vi "User Interface.vi"(10 "Test File Path":path=path "") -> ()   [LabVIEW 2020, in "Execution UI.lvclass"]
uses:
  Execution UI.lvclass
  Execution UI.lvclass/Execution UI.ctl
  Helper Classes/Test Tree/Test Tree.lvclass
  Helper Classes/Test Result Tree/Test Result Tree.lvclass
  Result Classes/Test Case Result/Test Case Result.lvclass
  Result Classes/Method Result/Method Result.lvclass
  Result Classes/Test Suite Result/Test Suite Result.lvclass
  Application Framework/Process Classes/Process/Process.lvclass
  Application Framework/Process Classes/Error Handler/Error Handler.lvclass
  <vilib>/Utility/miscctls.llb/LVNodeAndColumnTypeDef.ctl
  Test Runner/Test Runner.lvclass
  Private/TypeDefs/Execution State.ctl
  Helper Classes/Buffered Test Finder/Indexing Test Finder.lvclass
  Helper Classes/Result Table/Result Table/Result Table.lvclass
  Report Generator/Report Generator.lvclass
  Result Classes/Result View/Result View.vi
  Test Result View/Test Result View.lvclass
  Helper Classes/Test Finder/Test Finder.lvclass
  Execution Profiler/Execution Profiler.lvclass
  <vilib>/Platform/browser.llb/Open URL in Default Browser (string).vi
  Coverage Analyzer Process/Coverage Analyzer Process.lvclass
  C:/Git/astemes-lunit/source/Framework/Helper Classes/Test Tree/Test Tree.lvclass
  C:/Git/astemes-lunit/source/Framework/Helper Classes/Test Result Tree/Test Result Tree.lvclass
  C:/Git/astemes-lunit/source/Application Framework/Process Classes/Process/Process.lvclass
  C:/Git/astemes-lunit/source/Framework/Execution UI/Execution UI.lvclass
  C:/Git/astemes-lunit/source/Framework/Helper Classes/Test Finder/Test Finder.lvclass
  C:/Git/astemes-lunit/source/Framework/Helper Classes/Buffered Test Finder/Indexing Test Finder.lvclass
  C:/Git/astemes-lunit/source/Framework/Execution Profiler/Execution Profiler.lvclass
  C:/Git/astemes-lunit/source/Framework/Coverage Analyzer Process/Coverage Analyzer Process.lvclass
panel:
  in  "Refresh":bool
  in  "Run Single Test":bool
  in  "Stop":bool
  in  "Run All Tests":bool
  in  "Eject":bool
  in  "Save":bool
  in  "Collapse":bool
  in  "Expand":bool
  out "Progress bar":dbl(slide) scale=0.0..100.0
  out "Results":i32(listbox)=-1
  in  "Test Results":string[](tree)
  in  "Filter fails":bool
  out "Description":string
  out "Status":string
  out "error out":errorcluster
  in  "error in (no error)":errorcluster
  # "1"
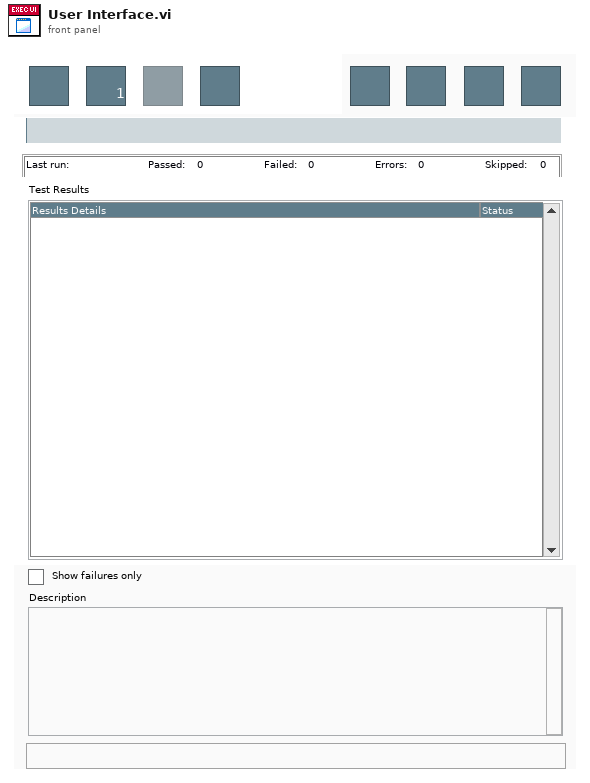
[diagram p1: front panel]
types:
  T1 = cluster{"Event Registration Refnum":refnum<event-registration>, "Event Registration Refnum":refnum<event-registration>, "Event Registration Refnum":refnum<event-registration>}
  T2 = typedef "LVNodeAndColumnTypeDef.ctl" = cluster{"Node":string, "Column":i32}
  T3 = enum32{"Invalid", "Standard", "Closed", "Hidden", "Minimized", "Maximized"}
  T4 = typedef "Execution UI.lvclass/Execution State.ctl" = enum16{"Idle", "Running"}
  T5 = enum8{"Enabled", "Disabled", "Disabled and Grayed Out"}
  T6 = typedef "Assertion Result.lvclass/Status.ctl" = enum16{"Pass", "Fail", "Error", "Skipped", "Setup Error", "Broken", "Teardown Error"}
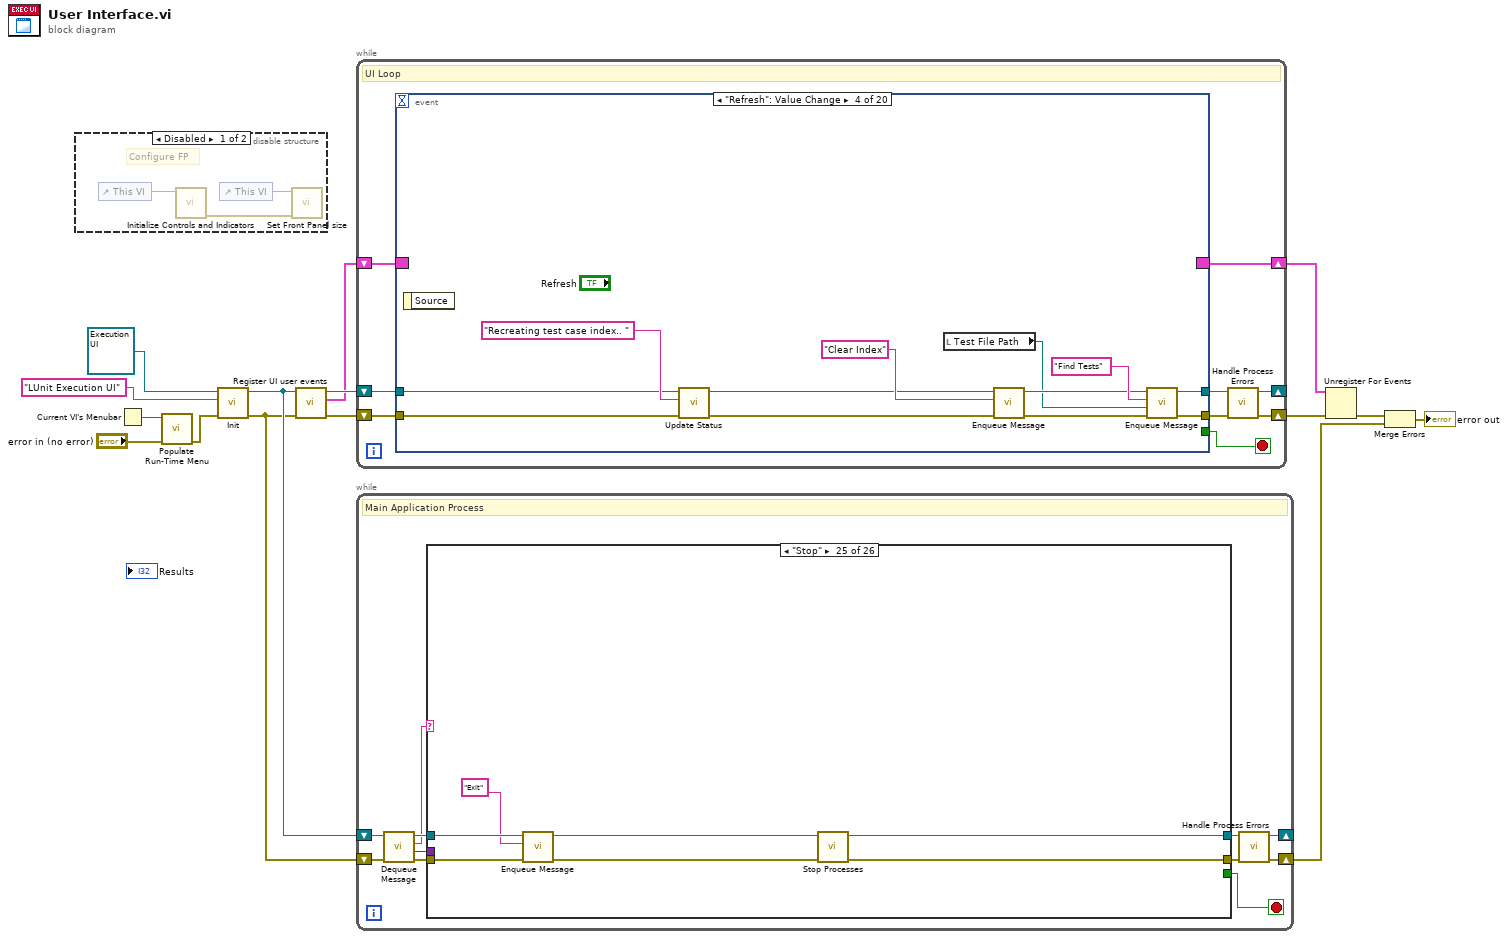
[diagram p0: block diagram]
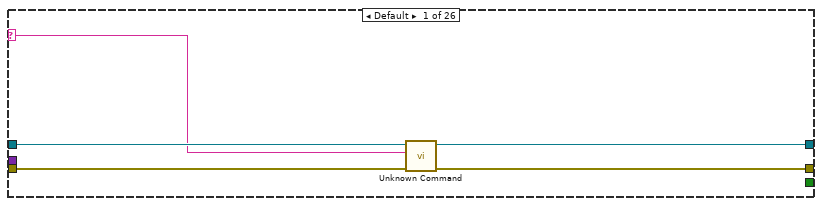
[diagram p2: hidden frame]
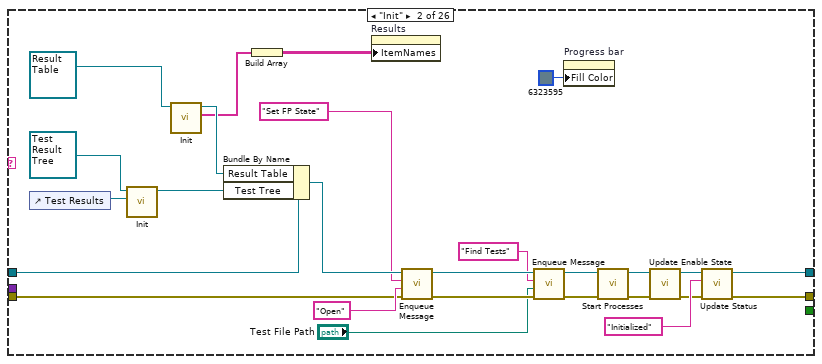
[diagram p3: hidden frame]
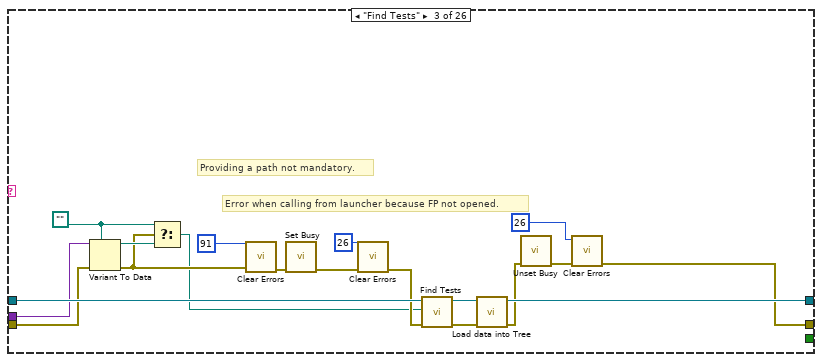
[diagram p4: hidden frame]
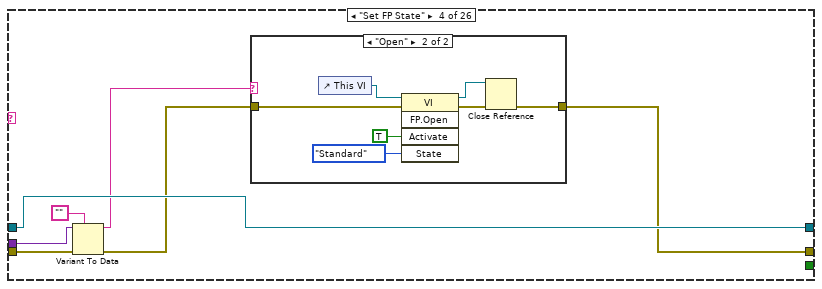
[diagram p5: hidden frame]
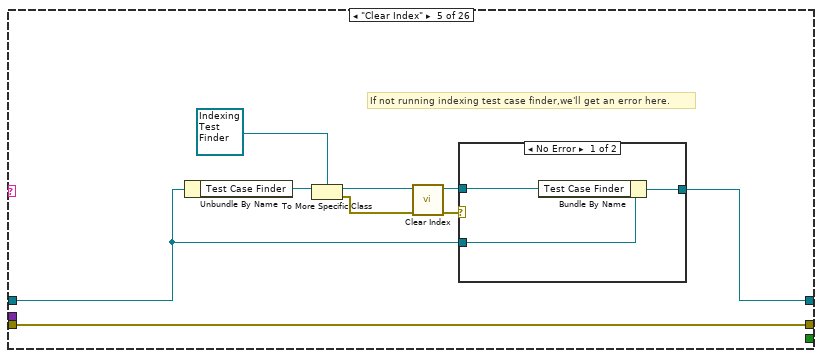
[diagram p7: hidden frame]
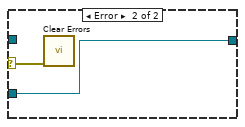
[diagram p8: hidden frame]
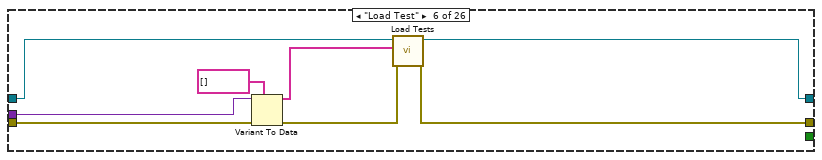
[diagram p9: hidden frame]
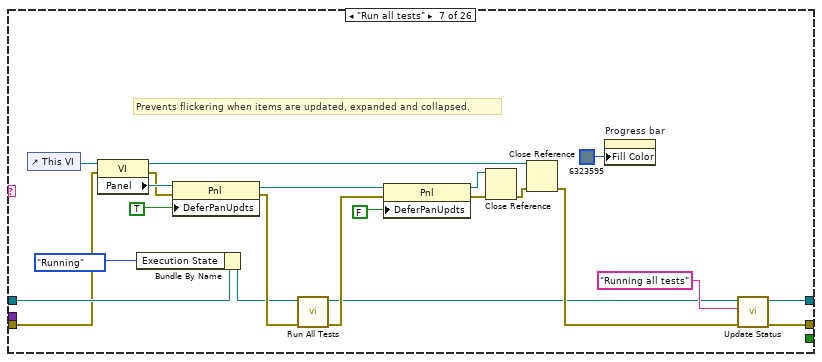
[diagram p10: hidden frame]
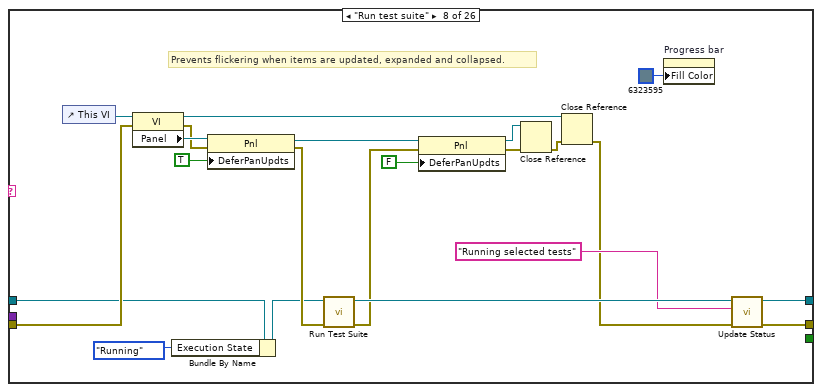
[diagram p11: hidden frame]
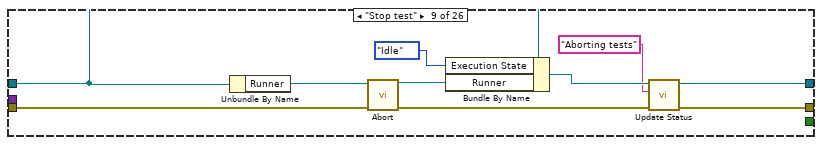
[diagram p12: hidden frame]
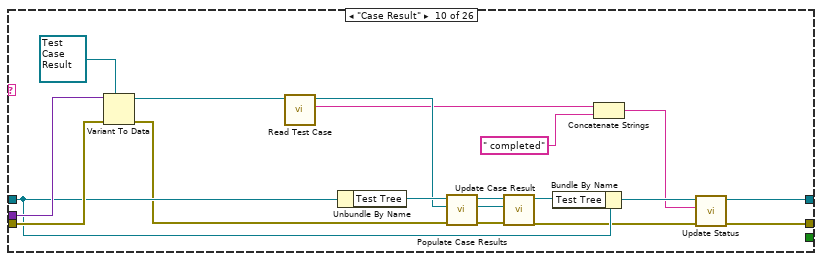
[diagram p13: hidden frame]
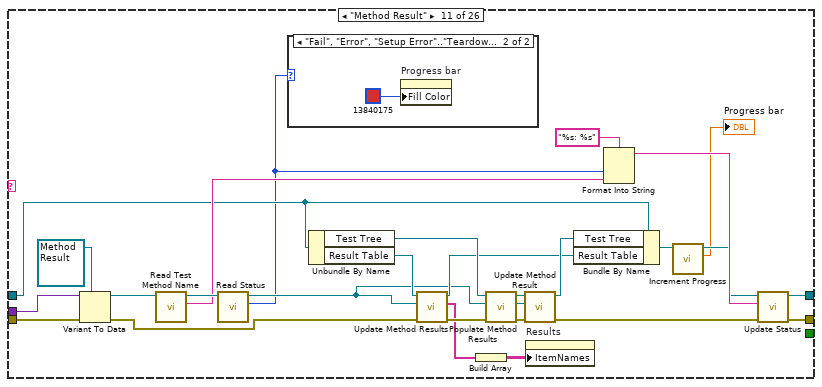
[diagram p14: hidden frame]
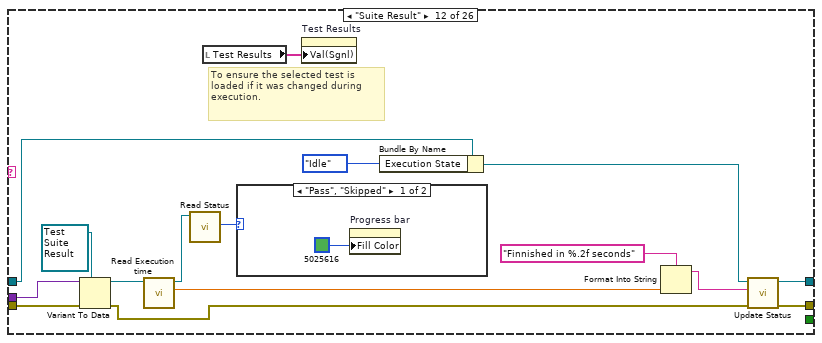
[diagram p16: hidden frame]
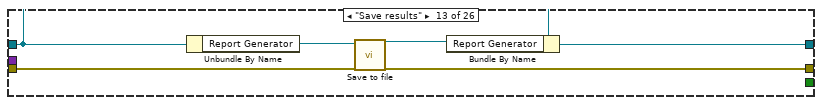
[diagram p18: hidden frame]
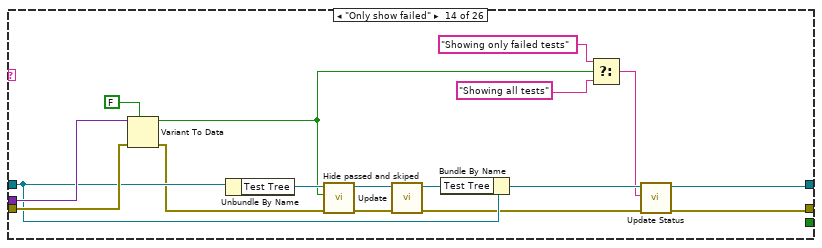
[diagram p19: hidden frame]
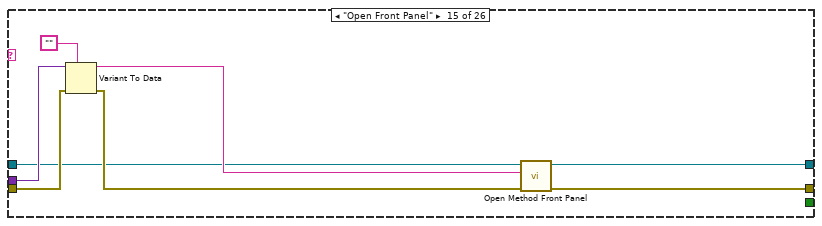
[diagram p20: hidden frame]
diagram:
  n1 = disable-structure shown="Disabled" {
    frame Disabled {
      # "Configure FP"
      n2 = control-ref of="This VI"() -> (w17:refnum<vi>)
      n3 = call "Initialize Controls and Indicators.vi"("VI in"=w17) -> ("error out"=w16:errorcluster)  [unwired: 10 in]
      n4 = control-ref of="This VI"() -> (w18:refnum<vi>)
      n5 = call "Set Front Panel size.vi"("error in (no error)"=w16, "VI in"=w18) -> ()  [unwired: 9 in, 1 out]
    }
    frame Enabled {
    }
  }
  n6 = Current VI's Menubar() -> (w1:refnum<k9>)
  n7 = call "Populate Run-Time Menu.vi"("error in (no error)"="error in (no error)", "Menu in"=w1) -> ("error out"=w2:errorcluster)  [unwired: 9 in]
  n8 = call-dynamic "Init.vi"("error in (no error)"=w2, "Name"="LUnit Execution UI", "Execution UI In"=refnum<class "Execution UI.lvclass"> refnum ("Test Execution UI.lvclass")) -> ("error out"=w7:errorcluster, "Execution UI Out"=w8:refnum<class "Execution UI.lvclass">)  [unwired: 7 in]
  n9 = call "Register UI user events.vi"("error in (no error)"=w7, "Execution UI In"=w8) -> ("error out"=w14:errorcluster, "output cluster"=w12:T1, "Execution UI Out"=w15:refnum<class "Execution UI.lvclass">)  [unwired: 7 in]
  n10 = while {
    shift-right: [w19] -> w6
    shift-left: w14 -> [w26]
    shift-right: [w21] -> _
    shift-left: w15 -> [w27]
    shift-right: [w23] -> w13
    shift-left: w12 -> [w22]
    stop <- w24 stop-if-true
    # "UI Loop"
    n11 = event shown="[3] \"Refresh\": Value Change" {
      selector: w22 -> [_ _ _ _ _ _ _ _ _ _ _ _ _ _ _ _ _ _ _ _]
      dyn-events: [_ _ _ _ _ _ _ _ _ _ _ _ _ _ _ _ _ _ _ _] -> w23
      timeout: _ -> [_ _ _ _ _ _ _ _ _ _ _ _ _ _ _ _ _ _ _ _]
      tunnel: w27 -> [w33 w36 w43 w47 w59 w69 w94 w101 w111 w116 w120 w130 w141 w149 w184 w305 w311 w312 w318 w326]
      tunnel: w26 -> [w34 w37 w41 w45 w61 w70 w96 w104 w110 w114 w118 w129 w131 w142 w183 w303 w309 w313 w320 w323]
      tunnel: [w34 w37 w40 w54 w58 w68 w93 w100 w108 w113 w119 w128 w132 w147 w182 w302 w308 w313 w317 w324] -> w20
      tunnel: [w33 w36 w42 w55 w56 w67 w91 w98 w109 w115 w121 w127 w141 w146 w181 w304 w310 w312 w315 w325] -> w25
      tunnel: [_ _ _ _ _ _ _ _ _ _ _ _ _ _ _ _ _ TRUE _ _] -> w24
      event "Collapse": Value Change {
        n12 = event-data() -> ()  [unwired: 1 in, 6 out]
        n13 = property on="Test Results" class="Tree (strict)"() -> ("All Tags"=w31:string[])  [unwired: 2 in, 2 out]
        n14 = invoke on="Test Results" class="Tree (strict)" method="Open/Close.Open/Close All"("Open"=FALSE ("Open?")) -> ()  [unwired: 3 in, 4 out]
        n15 = Index Array(array=w31) -> (element=w28:string)  [unwired: 1 in]
        n16 = Bundle By Name(cluster=T2 {"Node"="", "Column"=0} ("Top Left Visible Cell"), "Node"=w28) -> (w29:T2)
        n17 = property on="Test Results" class="Tree (strict)"("TopLeft"=w29) -> ()  [unwired: 2 in, 2 out]
      }
      event "Expand": Value Change {
        n18 = event-data() -> ()  [unwired: 1 in, 6 out]
        n19 = invoke on="Test Results" class="Tree (strict)" method="Open/Close.Open/Close All"("Open"=TRUE ("Open?")) -> ()  [unwired: 3 in, 4 out]
      }
      event "Filter fails": Value Change {
        n20 = event-data() -> ()  [unwired: 1 in, 1 out]
        n21 = call "Enqueue Message.vi"("error in (no error)"=w41, "Message Data"="Filter fails", "Message"="Only show failed", "Process In"=w43) -> ("error out"=w40:errorcluster, "Process Out"=w42:refnum<class "Execution UI.lvclass">)  [unwired: 6 in]
      }
      event "Refresh": Value Change {
        n22 = event-data() -> ()  [unwired: 1 in, 1 out]
        n23 = call "Update Status.vi"("error in (no error)"=w45, "Status"="Recreating test case index.. ", "Execution UI In"=w47) -> ("error out"=w46:errorcluster, "Execution UI Out"=w48:refnum<class "Execution UI.lvclass">)  [unwired: 7 in]
        n24 = local read "Test File Path"() -> (w44:path)
        n25 = call "Enqueue Message.vi"("error in (no error)"=w46, "Message"="Clear Index", "Process In"=w48) -> ("error out"=w51:errorcluster, "Process Out"=w52:refnum<class "Execution UI.lvclass">)  [unwired: 7 in]
        n26 = call "Enqueue Message.vi"("error in (no error)"=w51, "Message Data"=w44, "Message"="Find Tests", "Process In"=w52) -> ("error out"=w54:errorcluster, "Process Out"=w55:refnum<class "Execution UI.lvclass">)  [unwired: 6 in]
      }
      event "Run All Tests": Value Change {
        w60 = "Run all tests"  # Message
        n27 = event-data() -> ()  [unwired: 1 in, 1 out]
        n28 = call "Enqueue Message.vi"("error in (no error)"=w61, "Message"=w60, "Process In"=w59) -> ("error out"=w62:errorcluster, "Process Out"=w57:refnum<class "Execution UI.lvclass">)  [unwired: 7 in]
        n29 = call "Update Enable State.vi"("error in (no error)"=w62, "Execution UI In"=w57) -> ("error out"=w58:errorcluster, "Execution UI Out"=w56:refnum<class "Execution UI.lvclass">)  [unwired: 8 in]
      }
      event Key Down {
        # "Run all tests on ctrl+r"
        n30 = event-data() -> ("Char"=w63:i16, "PlatMods.Ctrl"=w66:bool, "PlatMods.Opt"=w65:bool)  [unwired: 1 in]
        n31 = Or(x=w66, y=w65) -> (x .or. y?=w64:bool)
        n32 = case "CTRL" shown="True" w64 {
          tunnel: w70 -> [w71 w77]
          tunnel: w69 -> [w72 w76]
          tunnel: [w71 w75] -> w68
          tunnel: [w72 w74] -> w67
          tunnel: w63 -> [_ w73]
          frame False {
          }
          frame True {
            n33 = case "Key" shown="119" w73 {
              tunnel: w77 -> [w78 w85 w89]
              tunnel: w76 -> [w79 w83 w90]
              tunnel: [w78 w82 w87] -> w75
              tunnel: [w79 w80 w88] -> w74
              frame Default {
              }
              frame 114 {
                w84 = "Run all tests"  # Message
                # "R"
                n34 = call "Enqueue Message.vi"("error in (no error)"=w85, "Message"=w84, "Process In"=w83) -> ("error out"=w86:errorcluster, "Process Out"=w81:refnum<class "Execution UI.lvclass">)  [unwired: 7 in]
                n35 = call "Update Enable State.vi"("error in (no error)"=w86, "Execution UI In"=w81) -> ("error out"=w82:errorcluster, "Execution UI Out"=w80:refnum<class "Execution UI.lvclass">)  [unwired: 8 in]
              }
              frame 119 {
                # "W"
                n36 = call-dynamic "Stop.vi"("error in (no error)"=w89, "Execution UI In"=w90) -> ("error out"=w87:errorcluster, "Execution UI Out"=w88:refnum<class "Execution UI.lvclass">)  [unwired: 7 in, 1 out]
              }
            }
          }
        }
      }
      event "Run Single Test": Value Change {
        w95 = "Run test suite"  # Message
        n37 = event-data() -> ()  [unwired: 1 in, 1 out]
        n38 = call "Enqueue Message.vi"("error in (no error)"=w96, "Message"=w95, "Process In"=w94) -> ("error out"=w97:errorcluster, "Process Out"=w92:refnum<class "Execution UI.lvclass">)  [unwired: 7 in]
        n39 = call "Update Enable State.vi"("error in (no error)"=w97, "Execution UI In"=w92) -> ("error out"=w93:errorcluster, "Execution UI Out"=w91:refnum<class "Execution UI.lvclass">)  [unwired: 8 in]
      }
      event "Stop": Value Change {
        n40 = event-data() -> ()  [unwired: 1 in, 2 out]
        n41 = call "Enqueue Message.vi"("error in (no error)"=w104, "Message"="Stop test", "Process In"=w101) -> ("error out"=w103:errorcluster, "Process Out"=w99:refnum<class "Execution UI.lvclass">)  [unwired: 7 in]
        n42 = call "Update Enable State.vi"("error in (no error)"=w103, "Execution UI In"=w99) -> ("error out"=w100:errorcluster, "Execution UI Out"=w98:refnum<class "Execution UI.lvclass">)  [unwired: 8 in]
      }
      event "Test Results": Double Click {
        n43 = event-data() -> ("Tag"=w106:string)  [unwired: 1 in]
        n44 = To Variant(anything=w106) -> (Variant=w105:variant)
        n45 = call "Enqueue Message.vi"("error in (no error)"=w110, "Message Data"=w105, "Message"="Open Front Panel", "Process In"=w111) -> ("error out"=w108:errorcluster, "Process Out"=w109:refnum<class "Execution UI.lvclass">)  [unwired: 6 in]
      }
      event "Save": Value Change {
        n46 = event-data() -> ()  [unwired: 1 in, 4 out]
        n47 = call "Enqueue Message.vi"("error in (no error)"=w114, "Message"="Save results", "Process In"=w116) -> ("error out"=w113:errorcluster, "Process Out"=w115:refnum<class "Execution UI.lvclass">)  [unwired: 7 in]
      }
      event "Eject": Value Change {
        n48 = event-data() -> ()  [unwired: 1 in, 4 out]
        n49 = call "Enqueue Message.vi"("error in (no error)"=w118, "Message"="Launch Results View", "Process In"=w120) -> ("error out"=w119:errorcluster, "Process Out"=w121:refnum<class "Execution UI.lvclass">)  [unwired: 7 in]
      }
      event "Test Results": Value Change {
        n50 = event-data() -> ("NewVal"=w122:string[])  [unwired: 1 in]
        n51 = call "Enqueue Message.vi"("error in (no error)"=w129, "Message Data"=w122, "Message"="Update Description", "Process In"=w130) -> ("error out"=w126:errorcluster, "Process Out"=w125:refnum<class "Execution UI.lvclass">)  [unwired: 6 in]
        n52 = call "Enqueue Message.vi"("error in (no error)"=w126, "Message Data"=w122, "Message"="Load Test", "Process In"=w125) -> ("error out"=w128:errorcluster, "Process Out"=w127:refnum<class "Execution UI.lvclass">)  [unwired: 6 in]
      }
      event Pane Size {
        # "Set column sizes on pane resize."
        n53 = event-data() -> ()  [unwired: 1 in, 1 out]
        n54 = property on="Test Results" class="Tree (strict)"(error in=w131) -> (error out=w133:errorcluster, "Width"=w134:u32)  [unwired: 1 in, 1 out]
        n55 = Quotient & Remainder(x=w134, y=u32 10) -> (floor(x/y)=w138:u32)  [unwired: 1 out]
        n56 = Multiply(x=w138, y=u32 8) -> (x*y=w135:u32)
        n57 = property on="Test Results" class="Tree (strict)"(error in=w133, "ActiveColNum"=0 ("Active Cell:Active Column Number"), "Width"=w135, "ActiveColNum"=1 ("Active Cell:Active Column Number"), "Width"=w135) -> (error out=w132:errorcluster)  [unwired: 1 in, 1 out]
      }
      event "Test File Path": Value Change {
        # "This case is triggered when running test cases through VI Server.\nTo control test execution from an external VI - get a reference to the \"Test File Path\" control on the User Interface.vi and update the value with the path to test case using a property node."
        n58 = event-data() -> ("NewVal"=w148:path)  [unwired: 1 in]
        n59 = call <vilib>:"Get File Extension.vi"("error in (no error)"=w142, "file"=w148) -> ("error out"=w143:errorcluster, "lowercase file extension"=w144:string, "dup file"=w145:path)  [unwired: 5 in, 2 out]
        n60 = case shown="Default" w144 {
          tunnel: w149 -> [w151 w170 w179]
          tunnel: w143 -> [w150 w169 w178]
          tunnel: w145 -> [_ w164 w176]
          tunnel: [w150 w156 w173] -> w147
          tunnel: [w151 w154 w172] -> w146
          frame Default {
          }
          frame "lvclass" {
            n61 = call "Enqueue Message.vi"("error in (no error)"=w169, "Message Data"=w164, "Message"="Find Tests", "Process In"=w170) -> ("error out"=w160:errorcluster, "Process Out"=w162:refnum<class "Execution UI.lvclass">)  [unwired: 6 in]
            n62 = call <vilib>:"Get LV Class Default Value.vi"("error in (no error)"=w160, "class path"=w164) -> ("error out"=w166:errorcluster, "object"=w165:refnum<class>)  [unwired: 8 in]
            n63 = call <vilib>:"Get LV Class Name.vi"("error in (no error)"=w166, "object"=w165) -> ("error out"=w159:errorcluster, "class name"=w153:string)  [unwired: 8 in]
            n64 = Build Array(w153) -> (w158:string[])
            n65 = call "Enqueue Message.vi"("error in (no error)"=w159, "Message Data"=w158, "Message"="Load Test", "Process In"=w162) -> ("error out"=w163:errorcluster, "Process Out"=w161:refnum<class "Execution UI.lvclass">)  [unwired: 6 in]
            n66 = call "Enqueue Message.vi"("error in (no error)"=w163, "Message"="Run test suite", "Process In"=w161) -> ("error out"=w157:errorcluster, "Process Out"=w155:refnum<class "Execution UI.lvclass">)  [unwired: 7 in]
            n67 = call "Enqueue Message.vi"("error in (no error)"=w157, "Message Data"=w153, "Message"="Set Top Left Tree Node", "Process In"=w155) -> ("error out"=w156:errorcluster, "Process Out"=w154:refnum<class "Execution UI.lvclass">)  [unwired: 6 in]
          }
          frame "lvproj" {
            n68 = call "Enqueue Message.vi"("error in (no error)"=w178, "Message Data"=w176, "Message"="Find Tests", "Process In"=w179) -> ("error out"=w174:errorcluster, "Process Out"=w175:refnum<class "Execution UI.lvclass">)  [unwired: 6 in]
            n69 = call "Enqueue Message.vi"("error in (no error)"=w174, "Message"="Run all tests", "Process In"=w175) -> ("error out"=w173:errorcluster, "Process Out"=w172:refnum<class "Execution UI.lvclass">)  [unwired: 7 in]
          }
        }
      }
      event Menu Selection (User) {
        n70 = event-data() -> ("ItemTag"=w185:string)  [unwired: 1 in]
        n71 = case shown="\"Coverage Analyzer...\"" w185 {
          tunnel: w184 -> [w199 w201 w208 w223 w226 w238 w255 w268 w272 w277 w285 w289 w293 w294 w299]
          tunnel: w183 -> [w186 w200 w209 w224 w227 w235 w252 w270 w276 w281 w282 w286 w290 w295 w298]
          tunnel: [w187 w200 w210 w221 w228 w236 w253 w269 w274 w279 w283 w287 w291 w295 w297] -> w182
          tunnel: [w199 w201 w211 w220 w229 w237 w254 w268 w273 w278 w285 w289 w293 w294 w296] -> w181
          frame "Full size" {
            # "This is the same as done in event case for Result Pane: Pane Size, but that case is not trigerd on maximizing window."
            n72 = control-ref of="This VI"() -> (w198:refnum<vi>)
            n73 = property on="Property Node" class="VI"(reference=w198, error in=w186, "FP.State"=T3."Maximized" ("Front Panel Window:State")) -> (error out=w189:errorcluster)  [unwired: 1 out]
            n74 = property on="Test Results" class="Tree (strict)"(error in=w189) -> (error out=w188:errorcluster, "Width"=w196:u32)  [unwired: 1 in, 1 out]
            n75 = Quotient & Remainder(x=w196, y=u32 10) -> (floor(x/y)=w195:u32)  [unwired: 1 out]
            n76 = Multiply(x=w195, y=u32 7) -> (x*y=w194:u32)
            n77 = property on="Test Results" class="Tree (strict)"(error in=w188, "ActiveColNum"=0 ("Active Cell:Active Column Number"), "Width"=w194, "ActiveColNum"=1 ("Active Cell:Active Column Number"), "Width"=w194) -> (error out=w187:errorcluster)  [unwired: 1 in, 1 out]
          }
          frame Default {
          }
          frame "Open Project or Test class" {
            n78 = call "File Dialog"("prompt"="Please select a test class or project file to load.", "pattern (all files)"="*.lvclass;*.lvproj;*.lvlib", "pattern label"="Project or class") -> ("selected path"=w207:path, "cancelled"=w203:bool, "error out"=w202:errorcluster)  [unwired: 9 in, 1 out]
            n79 = call <vilib>:"Clear Errors.vi"("error in (no error)"=w202) -> ()  [unwired: 5 in, 2 out]
            n80 = case shown="False" w203 {
              tunnel: [w213 w219] -> w211
              tunnel: [w212 w218] -> w210
              tunnel: w209 -> [w212 w217]
              tunnel: w208 -> [w213 w216]
              tunnel: w207 -> [_ w215]
              frame True {
              }
              frame False {
                n81 = call "Enqueue Message.vi"("error in (no error)"=w217, "Message Data"=w215, "Message"="Find Tests", "Process In"=w216) -> ("error out"=w218:errorcluster, "Process Out"=w219:refnum<class "Execution UI.lvclass">)  [unwired: 6 in]
              }
            }
          }
          frame "Configure Test Runner" {
            n82 = Unbundle By Name(w223) -> ("Runner"=w225:refnum<class "Test Runner.lvclass">)
            n83 = call "Configure Test Runner.vi"("error in (no error)"=w224, "Report Generator In"=w225) -> ("error out"=w221:errorcluster, "Report Generator Out"=w222:refnum<class "Test Runner.lvclass">)  [unwired: 8 in]
            n84 = Bundle By Name(cluster=w223, "Runner"=w222) -> (w220:refnum<class "Execution UI.lvclass">)
          }
          frame "Configure Reporting" {
            n85 = Unbundle By Name(w226) -> ("Report Generator"=w231:refnum<class "Report Generator.lvclass">)
            n86 = call "Configure Report Generator.vi"("error in (no error)"=w227, "Report Generator In"=w231) -> ("error out"=w228:errorcluster, "Report Generator Out"=w230:refnum<class "Report Generator.lvclass">)  [unwired: 8 in]
            n87 = Bundle By Name(cluster=w226, "Report Generator"=w230) -> (w229:refnum<class "Execution UI.lvclass">)
          }
          frame "Execution Profiler..." {
            n88 = Current VI's Menubar() -> (w233:refnum<k9>)
            n89 = Get Menu Item Info(7:"Execution Profiler...", 11:w233) -> (4:w234:bool)  [unwired: 1 in, 6 out]
            n90 = case shown="False" w234 {
              tunnel: w238 -> [w243 w248]
              tunnel: [w242 w247] -> w237
              tunnel: [w241 w246] -> w236
              tunnel: w235 -> [w240 w245]
              frame False {
                n91 = call "Enqueue Message.vi"("error in (no error)"=w240, "Message"="Enable Execution Profiler", "Process In"=w243) -> ("error out"=w241:errorcluster, "Process Out"=w242:refnum<class "Execution UI.lvclass">)  [unwired: 7 in]
              }
              frame True {
                n92 = call "Enqueue Message.vi"("error in (no error)"=w245, "Message"="Disable Execution Profiler", "Process In"=w248) -> ("error out"=w246:errorcluster, "Process Out"=w247:refnum<class "Execution UI.lvclass">)  [unwired: 7 in]
              }
            }
          }
          frame "Coverage Analyzer..." {
            n93 = Current VI's Menubar() -> (w250:refnum<k9>)
            n94 = Get Menu Item Info(7:"Coverage Analyzer...", 11:w250) -> (4:w251:bool)  [unwired: 1 in, 6 out]
            n95 = case shown="True" w251 {
              tunnel: w255 -> [w260 w265]
              tunnel: [w259 w264] -> w254
              tunnel: [w258 w263] -> w253
              tunnel: w252 -> [w257 w262]
              frame False {
                n96 = call "Enqueue Message.vi"("error in (no error)"=w257, "Message"="Enable Coverage Analyzer", "Process In"=w260) -> ("error out"=w258:errorcluster, "Process Out"=w259:refnum<class "Execution UI.lvclass">)  [unwired: 7 in]
              }
              frame True {
                n97 = call "Enqueue Message.vi"("error in (no error)"=w262, "Message"="Disable Coverage Analyzer", "Process In"=w265) -> ("error out"=w263:errorcluster, "Process Out"=w264:refnum<class "Execution UI.lvclass">)  [unwired: 7 in]
              }
            }
          }
          frame "Reset..." {
            n98 = control-ref of="This VI"() -> (w266:refnum<vi>)
            n99 = call "Initialize Controls and Indicators.vi"("error in (no error)"=w270, "VI in"=w266) -> ("error out"=w271:errorcluster)  [unwired: 9 in]
            n100 = control-ref of="This VI"() -> (w267:refnum<vi>)
            n101 = call "Set Front Panel size.vi"("error in (no error)"=w271, "VI in"=w267) -> ("error out"=w269:errorcluster)  [unwired: 9 in]
          }
          frame "New Test Case" {
            # "Not implemented."
            n102 = call "Enqueue Message.vi"("error in (no error)"=w276, "Message"="Find Tests", "Process In"=w272) -> ("error out"=w274:errorcluster, "Process Out"=w273:refnum<class "Execution UI.lvclass">)  [unwired: 7 in]
          }
          frame "New Test Vector" {
            # "Not implemented."
            n103 = call "Enqueue Message.vi"("error in (no error)"=w281, "Message"="Find Tests", "Process In"=w277) -> ("error out"=w279:errorcluster, "Process Out"=w278:refnum<class "Execution UI.lvclass">)  [unwired: 7 in]
          }
          frame "Documentation..." {
            n104 = call-poly <vilib>:"Open URL in Default Browser.vi"("error in (no error)"=w282, "URL"="https://astemes.github.io/astemes-lunit/") -> ("error out"=w283:errorcluster)  [unwired: 4 in, 1 out]
          }
          frame "Report issue..." {
            n105 = call-poly <vilib>:"Open URL in Default Browser.vi"("error in (no error)"=w286, "URL"="https://github.com/astemes/astemes-lunit/issues") -> ("error out"=w287:errorcluster)  [unwired: 4 in, 1 out]
          }
          frame "Post an Idea..." {
            n106 = call-poly <vilib>:"Open URL in Default Browser.vi"("error in (no error)"=w290, "URL"="https://www.vipm.io/post/suggestion/?package_name=astemes_lib_lunit&return_url=/package/astemes_lib_lunit/") -> ("error out"=w291:errorcluster)  [unwired: 4 in, 1 out]
          }
          frame "About" {
            n107 = call "About Dialog.vi"() -> ()  [unwired: 12 in]
          }
          frame "Exit" {
            n108 = call-dynamic "Stop.vi"("error in (no error)"=w298, "Execution UI In"=w299) -> ("error out"=w297:errorcluster, "Execution UI Out"=w296:refnum<class "Execution UI.lvclass">)  [unwired: 7 in, 1 out]
          }
        }
      }
      event User Event {
        n109 = event-data() -> ("Case Result"=w300:refnum<class "Test Case Result.lvclass">)  [unwired: 1 in]
        n110 = call "Enqueue Message.vi"("error in (no error)"=w303, "Message Data"=w300, "Message"="Case Result", "Process In"=w305) -> ("error out"=w302:errorcluster, "Process Out"=w304:refnum<class "Execution UI.lvclass">)  [unwired: 6 in]
      }
      event User Event {
        n111 = event-data() -> ("Method Result"=w306:refnum<class "Method Result.lvclass">)  [unwired: 1 in]
        n112 = call "Enqueue Message.vi"("error in (no error)"=w309, "Message Data"=w306, "Message"="Method result", "Process In"=w311) -> ("error out"=w308:errorcluster, "Process Out"=w310:refnum<class "Execution UI.lvclass">)  [unwired: 6 in]
      }
      event User Event {
        n113 = event-data() -> ()  [unwired: 1 in, 4 out]
      }
      event User Event {
        n114 = event-data() -> ("Suite Result"=w321:refnum<class "Test Suite Result.lvclass">)  [unwired: 1 in]
        n115 = call "Enqueue Message.vi"("error in (no error)"=w320, "Message Data"=w321, "Message"="Suite Result", "Process In"=w318) -> ("error out"=w319:errorcluster, "Process Out"=w316:refnum<class "Execution UI.lvclass">)  [unwired: 6 in]
        n116 = call "Update Enable State.vi"("error in (no error)"=w319, "Execution UI In"=w316) -> ("error out"=w317:errorcluster, "Execution UI Out"=w315:refnum<class "Execution UI.lvclass">)  [unwired: 8 in]
      }
      event Panel Close? {
        w327 = TRUE  # Discard?
        n117 = event-data() -> ()  [unwired: 1 in, 4 out]
        n118 = call-dynamic "Stop.vi"("error in (no error)"=w323, "Execution UI In"=w326) -> ("error out"=w324:errorcluster, "Execution UI Out"=w325:refnum<class "Execution UI.lvclass">)  [unwired: 7 in, 1 out]
        n119 = event-data ("Event Filter Node")("Discard?"=w327) -> ()  [unwired: 1 in, 1 out]
      }
    }
    n120 = call "Handle Process Errors.vi"("error in (no error)"=w20, "Process In"=w25) -> ("error out"=w19:errorcluster, "Process Out"=w21:refnum<class "Execution UI.lvclass">)  [unwired: 8 in]
  }
  n121 = while {
    shift-right: [w329] -> w10
    shift-left: w7 -> [w337]
    shift-right: [w330] -> _
    shift-left: w8 -> [w338]
    stop <- w333 stop-if-true
    # "Main Application Process"
    n122 = call "Dequeue Message.vi"("error in (no error)"=w337, "Process In"=w338) -> ("error out"=w335:errorcluster, "Message Data"=w331:variant, "Message"=w332:string, "Process Out"=w336:refnum<class "Execution UI.lvclass">)  [unwired: 6 in]
    n123 = case shown="\"Stop\"" w332 {
      selector: w332 -> [w339 _ _ _ _ _ _ _ _ _ _ _ _ _ _ _ _ _ _ _ _ _ _ _ _ _]
      tunnel: w336 -> [w340 w365 w388 w395 w412 w425 w447 w449 w476 w495 w516 w534 w550 w565 w568 w578 w602 w606 w617 w645 w664 w681 w695 w709 w715 w724]
      tunnel: [w341 w348 w384 w395 w406 w424 w446 w468 w470 w489 w523 w539 w547 w557 w572 w578 w597 w606 w617 w645 w662 w679 w693 w707 w712 w728] -> w334
      tunnel: w335 -> [w342 w344 w379 w393 w404 w420 w439 w450 w475 w498 w526 w543 w548 w567 w575 w584 w603 w609 w618 w643 w647 w677 w690 w704 w716 w718]
      tunnel: [w343 w347 w371 w394 w404 w419 w445 w467 w473 w488 w522 w538 w545 w555 w571 w579 w594 w605 w618 w644 w663 w680 w694 w708 w711 w727] -> w328
      tunnel: [_ _ _ _ _ _ _ _ _ _ _ _ _ _ _ _ _ _ _ _ _ _ _ _ _ TRUE] -> w333
      tunnel: w331 -> [_ _ w382 w391 _ w423 _ _ _ w497 w525 w542 _ w566 w574 w583 w601 w608 _ _ _ _ _ _ _ _]
      frame Default {
        n124 = call "Unknown Command.vi"("error in (no error)"=w342, "String"=w339, "Process In"=w340) -> ("error out"=w343:errorcluster, "Process Out"=w341:refnum<class "Execution UI.lvclass">)  [unwired: 7 in]
      }
      frame "Init" {
        n125 = control-ref of="Test Results"() -> (w368:refnum<vi>)
        n126 = call-dynamic "Init.vi"("Test Tree reference"=w368, "Test Tree In"=refnum<class "Test Result Tree.lvclass"> refnum ("Test Result Tree.lvclass")) -> ("Test Tree Out"=w366:refnum<class "Test Result Tree.lvclass">)  [unwired: 8 in, 1 out]
        n127 = call "Init.vi"("Result Table in"=refnum<class "Result Table.lvclass"> refnum) -> ("Result Texts"=w353:string[], "Result Table out"=w363:refnum<class "Result Table.lvclass">)  [unwired: 8 in, 1 out]
        n128 = Bundle By Name(cluster=w365, "Result Table"=w363, "Test Tree"=w366) -> (w362:refnum<class "Execution UI.lvclass">)
        n129 = Build Array(w353) -> (w352:string[][])
        n130 = property on="Results" class="MCListbox (strict)"("ItemNames"=w352) -> ()  [unwired: 2 in, 2 out]
        n131 = call "Enqueue Message.vi"("error in (no error)"=w344, "Message Data"="Open", "Message"="Set FP State", "Process In"=w362) -> ("error out"=w361:errorcluster, "Process Out"=w360:refnum<class "Execution UI.lvclass">)  [unwired: 6 in]
        n132 = call "Enqueue Message.vi"("error in (no error)"=w361, "Message Data"="Test File Path", "Message"="Find Tests", "Process In"=w360) -> ("error out"=w349:errorcluster, "Process Out"=w350:refnum<class "Execution UI.lvclass">)  [unwired: 6 in]
        n133 = property on="Progress bar" class="Slide (strict)"("Fill Color"=u32 6323595) -> ()  [unwired: 2 in, 2 out]
        n134 = call "Start Processes.vi"("error in (no error)"=w349, "Execution UI In"=w350) -> ("error out"=w357:errorcluster, "Execution UI Out"=w355:refnum<class "Execution UI.lvclass">)  [unwired: 8 in]
        n135 = call "Update Enable State.vi"("error in (no error)"=w357, "Execution UI In"=w355) -> ("error out"=w356:errorcluster, "Execution UI Out"=w354:refnum<class "Execution UI.lvclass">)  [unwired: 8 in]
        n136 = call "Update Status.vi"("error in (no error)"=w356, "Status"="Initialized", "Execution UI In"=w354) -> ("error out"=w347:errorcluster, "Execution UI Out"=w348:refnum<class "Execution UI.lvclass">)  [unwired: 7 in]
      }
      frame "Find Tests" {
        w381 = path "" ("Not A Path Constant")
        # "Error when calling from launcher because FP not opened."
        # "Providing a path not mandatory."
        n137 = Variant To Data(error in=w379, type=w381, Variant=w382) -> (data=w380:path, error out=w376:errorcluster)
        n138 = Select(t=w381, s=w376, f=w380) -> (s? t:f=w370:path)
        n139 = call <vilib>:"Clear Errors.vi"("error in (no error)"=w376, "specific error code to clear (0: all)"=91) -> ("error out"=w378:errorcluster)  [unwired: 4 in, 1 out]
        n140 = call <vilib>:"Set Busy.vi"("error in (no error)"=w378) -> ("error out"=w387:errorcluster)  [unwired: 9 in, 1 out]
        n141 = call <vilib>:"Clear Errors.vi"("error in (no error)"=w387, "specific error code to clear (0: all)"=26) -> ("error out"=w375:errorcluster)  [unwired: 4 in, 1 out]
        n142 = call "Find Tests.vi"("error in (no error)"=w375, "Project or Class Path"=w370, "Execution UI In"=w388) -> ("error out"=w383:errorcluster, "Execution UI Out"=w385:refnum<class "Execution UI.lvclass">)  [unwired: 7 in]
        n143 = call "Load data into Tree.vi"("error in (no error)"=w383, "Execution UI In"=w385) -> ("error out"=w372:errorcluster, "Execution UI Out"=w384:refnum<class "Execution UI.lvclass">)  [unwired: 8 in]
        n144 = call <vilib>:"Unset Busy.vi"("error in (no error)"=w372) -> ("error out"=w386:errorcluster)  [unwired: 10 in]
        n145 = call <vilib>:"Clear Errors.vi"("error in (no error)"=w386, "specific error code to clear (0: all)"=26) -> ("error out"=w371:errorcluster)  [unwired: 4 in, 1 out]
      }
      frame "Set FP State" {
        n146 = Variant To Data(error in=w393, type="" ("Empty String Constant"), Variant=w391) -> (data=w389:string, error out=w392:errorcluster)
        n147 = case shown="\"Open\"" w389 {
          tunnel: [w396 w398] -> w394
          tunnel: w392 -> [w396 w397]
          frame Default {
          }
          frame "Open" {
            n148 = control-ref of="This VI"() -> (w401:refnum<vi>)
            n149 = invoke on="Invoke Node" class="VI" method="FP.Open"(reference=w401, error in=w397, "Activate"=TRUE ("Activate?"), "State"=T3."Standard") -> (reference out=w399:refnum<vi>, error out=w400:errorcluster)  [unwired: 1 in, 3 out]
            n150 = Close Reference(reference=w399, error in (no error)=w400) -> (error out=w398:errorcluster)
          }
        }
      }
      frame "Clear Index" {
        # "If not running indexing test case finder,we'll get an error here."
        n151 = Unbundle By Name(w412) -> ("Test Case Finder"=w411:refnum<class "Test Finder.lvclass">)
        n152 = To More Specific Class(target class=refnum<class "Indexing Test Finder.lvclass"> refnum ("Indexing Test Finder.lvclass"), reference=w411) -> (specific class reference=w410:refnum<class "Indexing Test Finder.lvclass">, error out=w408:errorcluster)  [unwired: 1 in]
        n153 = call "Clear Index.vi"("error in (no error)"=w408, "Indexing Test Finder in"=w410) -> ("error out"=w407:errorcluster, "Indexing Test Finder out"=w405:refnum<class "Indexing Test Finder.lvclass">)  [unwired: 8 in]
        n154 = case shown="No Error" w407 {
          selector: w407 -> [_ w416]
          tunnel: w412 -> [w415 w417]
          tunnel: [w414 w417] -> w406
          tunnel: w405 -> [w413 _]
          frame No Error {
            n155 = Bundle By Name(cluster=w415, "Test Case Finder"=w413) -> (w414:refnum<class "Execution UI.lvclass">)
          }
          frame Error {
            n156 = call <vilib>:"Clear Errors.vi"("error in (no error)"=w416) -> ()  [unwired: 5 in, 2 out]
          }
        }
      }
      frame "Load Test" {
        n157 = Variant To Data(error in=w420, type=string[] [], Variant=w423) -> (data=w418:string[], error out=w421:errorcluster)
        n158 = call "Load Tests.vi"("error in (no error)"=w421, "Tests"=w418, "Execution UI In"=w425) -> ("error out"=w419:errorcluster, "Execution UI Out"=w424:refnum<class "Execution UI.lvclass">)  [unwired: 7 in]
      }
      frame "Run all tests" {
        # "Prevents flickering when items are updated, expanded and collapsed."
        n159 = control-ref of="This VI"() -> (w443:refnum<vi>)
        n160 = property on="Property Node" class="VI"(reference=w443, error in=w439) -> (reference out=w433:refnum<vi>, error out=w441:errorcluster, "Panel"=w442:refnum<vi>)
        n161 = Bundle By Name(cluster=w447, "Execution State"=Execution_State."Running") -> (w429:refnum<class "Execution UI.lvclass">)
        n162 = property on="Property Node" class="Pnl"(reference=w442, error in=w441, "DeferPanUpdts"=TRUE ("Defer Panel Updates")) -> (reference out=w434:refnum<vi>, error out=w440:errorcluster)
        n163 = call "Run All Tests.vi"("error in (no error)"=w440, "Execution UI In"=w429) -> ("error out"=w432:errorcluster, "Execution UI Out"=w427:refnum<class "Execution UI.lvclass">)  [unwired: 8 in]
        n164 = property on="Property Node" class="Pnl"(reference=w434, error in=w432, "DeferPanUpdts"=FALSE ("Defer Panel Updates")) -> (reference out=w435:refnum<vi>, error out=w437:errorcluster)
        n165 = Close Reference(reference=w435, error in (no error)=w437) -> (error out=w436:errorcluster)
        n166 = Close Reference(reference=w433, error in (no error)=w436) -> (error out=w431:errorcluster)
        n167 = property on="Progress bar" class="Slide (strict)"("Fill Color"=u32 6323595) -> ()  [unwired: 2 in, 2 out]
        n168 = call "Update Status.vi"("error in (no error)"=w431, "Status"="Running all tests", "Execution UI In"=w427) -> ("error out"=w445:errorcluster, "Execution UI Out"=w446:refnum<class "Execution UI.lvclass">)  [unwired: 7 in]
      }
      frame "Run test suite" {
        # "Prevents flickering when items are updated, expanded and collapsed."
        n169 = control-ref of="This VI"() -> (w465:refnum<vi>)
        n170 = property on="Property Node" class="VI"(reference=w465, error in=w450) -> (reference out=w457:refnum<vi>, error out=w463:errorcluster, "Panel"=w464:refnum<vi>)
        n171 = Bundle By Name(cluster=w449, "Execution State"=Execution_State."Running") -> (w452:refnum<class "Execution UI.lvclass">)
        n172 = property on="Property Node" class="Pnl"(reference=w464, error in=w463, "DeferPanUpdts"=TRUE ("Defer Panel Updates")) -> (reference out=w458:refnum<vi>, error out=w455:errorcluster)
        n173 = call "Run Test Suite.vi"("error in (no error)"=w455, "Execution UI In"=w452) -> ("error out"=w454:errorcluster, "Execution UI Out"=w469:refnum<class "Execution UI.lvclass">)  [unwired: 8 in]
        n174 = property on="Property Node" class="Pnl"(reference=w458, error in=w454, "DeferPanUpdts"=FALSE ("Defer Panel Updates")) -> (reference out=w459:refnum<vi>, error out=w461:errorcluster)
        n175 = Close Reference(reference=w459, error in (no error)=w461) -> (error out=w460:errorcluster)
        n176 = Close Reference(reference=w457, error in (no error)=w460) -> (error out=w453:errorcluster)
        n177 = property on="Progress bar" class="Slide (strict)"("Fill Color"=u32 6323595) -> ()  [unwired: 2 in, 2 out]
        n178 = call "Update Status.vi"("error in (no error)"=w453, "Status"="Running selected tests", "Execution UI In"=w469) -> ("error out"=w467:errorcluster, "Execution UI Out"=w468:refnum<class "Execution UI.lvclass">)  [unwired: 7 in]
      }
      frame "Stop test" {
        n179 = Unbundle By Name(w476) -> ("Runner"=w479:refnum<class "Test Runner.lvclass">)
        n180 = call "Abort.vi"("error in (no error)"=w475, "Test Runner In"=w479) -> ("error out"=w474:errorcluster, "Test Runner Out"=w478:refnum<class "Test Runner.lvclass">)  [unwired: 8 in]
        n181 = Bundle By Name(cluster=w476, "Execution State"=Execution_State."Idle", "Runner"=w478) -> (w477:refnum<class "Execution UI.lvclass">)
        n182 = call "Update Status.vi"("error in (no error)"=w474, "Status"="Aborting tests", "Execution UI In"=w477) -> ("error out"=w473:errorcluster, "Execution UI Out"=w470:refnum<class "Execution UI.lvclass">)  [unwired: 7 in]
      }
      frame "Case Result" {
        n183 = Variant To Data(error in=w498, type=refnum<class "Test Case Result.lvclass"> refnum ("Case Result"), Variant=w497) -> (data=w485:refnum<class "Test Case Result.lvclass">, error out=w480:errorcluster)
        n184 = call "Read Test Case.vi"("Test Case Result In"=w485) -> ("Test Case"=w482:string, "Test Case Result Out"=w484:refnum<class "Test Case Result.lvclass">)  [unwired: 9 in]
        n185 = Unbundle By Name(w495) -> ("Test Tree"=w494:refnum<class "Test Result Tree.lvclass">)
        n186 = call "Populate Case Results.vi"("error in (no error)"=w480, "Test Case Result"=w484, "Test Tree In"=w494) -> ("error out"=w490:errorcluster, "Test Case Result Out out"=w481:refnum<class "Test Case Result.lvclass">, "Test Tree Out"=w492:refnum<class "Test Result Tree.lvclass">)  [unwired: 6 in]
        n187 = call "Update Case Result.vi"("error in (no error)"=w490, "Test Method Result"=w481, "Test Tree In"=w492) -> ("error out"=w487:errorcluster, "Test Tree Out"=w491:refnum<class "Test Result Tree.lvclass">)  [unwired: 7 in]
        n188 = Bundle By Name(cluster=w495, "Test Tree"=w491) -> (w493:refnum<class "Execution UI.lvclass">)
        n189 = Concatenate Strings(w482, " completed" ("Status")) -> (w483:string)
        n190 = call "Update Status.vi"("error in (no error)"=w487, "Status"=w483, "Execution UI In"=w493) -> ("error out"=w488:errorcluster, "Execution UI Out"=w489:refnum<class "Execution UI.lvclass">)  [unwired: 7 in]
      }
      frame "Method Result" {
        n191 = Variant To Data(error in=w526, type=refnum<class "Method Result.lvclass"> refnum ("Test Method Result.lvclass"), Variant=w525) -> (data=w517:refnum<class "Method Result.lvclass">, error out=w504:errorcluster)
        n192 = call "Read Test Method Name.vi"("Method Result In"=w517) -> ("Test Method Name"=w519:string, "Method Result Out"=w521:refnum<class "Method Result.lvclass">)  [unwired: 9 in]
        n193 = call "Read Status.vi"("Method Result In"=w521) -> ("Status"=w500:T6, "Method Result Out"=w501:refnum<class "Method Result.lvclass">)  [unwired: 8 in, 1 out]
        n194 = case shown="\"Fail\", \"Error\", \"Setup Error\"..\"Teardown Error\"" w500 {
          frame "Pass", "Skipped" {
          }
          frame "Fail", "Error", "Setup Error".."Teardown Error" {
            n195 = property on="Progress bar" class="Slide (strict)"("Fill Color"=u32 13840175) -> ()  [unwired: 2 in, 2 out]
          }
        }
        n196 = Unbundle By Name(w516) -> ("Test Tree"=w515:refnum<class "Test Result Tree.lvclass">, "Result Table"=w507:refnum<class "Result Table.lvclass">)
        n197 = call "Update Method Results.vi"("error in (no error)"=w504, "Method Result"=w501, "Result Table in"=w507) -> ("error out"=w505:errorcluster, "Result Texts"=w503:string[], "Result Table out"=w506:refnum<class "Result Table.lvclass">)  [unwired: 6 in]
        n198 = Build Array(w503) -> (w502:string[][])
        n199 = call "Populate Method Results.vi"("error in (no error)"=w505, "Test Method Result"=w501, "Test Tree In"=w515) -> ("error out"=w513:errorcluster, "Test Method Result Out"=w511:refnum<class "Method Result.lvclass">, "Test Tree Out"=w514:refnum<class "Test Result Tree.lvclass">)  [unwired: 6 in]
        n200 = call "Update Method Result.vi"("error in (no error)"=w513, "Test Method Result"=w511, "Test Tree In"=w514) -> ("error out"=w499:errorcluster, "Test Tree Out"=w512:refnum<class "Test Result Tree.lvclass">)  [unwired: 7 in]
        n201 = property on="Results" class="MCListbox (strict)"("ItemNames"=w502) -> ()  [unwired: 2 in, 2 out]
        n202 = Bundle By Name(cluster=w516, "Test Tree"=w512, "Result Table"=w506) -> (w510:refnum<class "Execution UI.lvclass">)
        n203 = Format Into String(format string="%s: %s", w500, w519) -> (resulting string=w518:string)  [unwired: 2 in, 1 out]
        n204 = call "Increment Progress.vi"("Execution UI In"=w510) -> ("Progress (%)"=→"Progress bar":dbl, "Execution UI Out"=w509:refnum<class "Execution UI.lvclass">)  [unwired: 9 in]
        n205 = call "Update Status.vi"("error in (no error)"=w499, "Status"=w518, "Execution UI In"=w509) -> ("error out"=w522:errorcluster, "Execution UI Out"=w523:refnum<class "Execution UI.lvclass">)  [unwired: 7 in]
      }
      frame "Suite Result" {
        # "To ensure the selected test is loaded if it was changed during execution."
        n206 = Variant To Data(error in=w543, type=refnum<class "Test Suite Result.lvclass"> refnum ("Test Suite Result.lvclass"), Variant=w542) -> (data=w540:refnum<class "Test Suite Result.lvclass">, error out=w530:errorcluster)
        n207 = call "Read Execution time.vi"("Test Suite Result In"=w540) -> ("Execution time"=w536:dbl, "Test Suite Result Out"=w529:refnum<class "Test Suite Result.lvclass">)  [unwired: 8 in, 1 out]
        n208 = call "Read Status.vi"("Test Suite Result In"=w529) -> ("Status"=w528:T6)  [unwired: 9 in, 1 out]
        n209 = local read "Test Results"() -> (w531:string[])
        n210 = case shown="\"Pass\", \"Skipped\"" w528 {
          frame "Pass", "Skipped" {
            n211 = property on="Progress bar" class="Slide (strict)"("Fill Color"=u32 5025616) -> ()  [unwired: 2 in, 2 out]
          }
          frame "Fail", "Error", "Setup Error".."Teardown Error" {
          }
        }
        n212 = property on="Test Results" class="Tree (strict)"("Val(Sgnl)"=w531) -> ()  [unwired: 2 in, 2 out]
        n213 = Bundle By Name(cluster=w534, "Execution State"=Execution_State."Idle") -> (w533:refnum<class "Execution UI.lvclass">)
        n214 = Format Into String(format string="Finnished in %.2f seconds", w536) -> (resulting string=w535:string)  [unwired: 2 in, 1 out]
        n215 = call "Update Status.vi"("error in (no error)"=w530, "Status"=w535, "Execution UI In"=w533) -> ("error out"=w538:errorcluster, "Execution UI Out"=w539:refnum<class "Execution UI.lvclass">)  [unwired: 7 in]
      }
      frame "Save results" {
        n216 = Unbundle By Name(w550) -> ("Report Generator"=w549:refnum<class "Report Generator.lvclass">)
        n217 = call "Save to file.vi"("error in (no error)"=w548, "Report Generator In"=w549) -> ("error out"=w545:errorcluster, "Report Generator Out"=w546:refnum<class "Report Generator.lvclass">)  [unwired: 8 in]
        n218 = Bundle By Name(cluster=w550, "Report Generator"=w546) -> (w547:refnum<class "Execution UI.lvclass">)
      }
      frame "Only show failed" {
        n219 = Variant To Data(error in=w567, type=FALSE, Variant=w566) -> (data=w551:bool, error out=w559:errorcluster)
        n220 = Unbundle By Name(w565) -> ("Test Tree"=w561:refnum<class "Test Result Tree.lvclass">)
        n221 = call "Hide passed and skiped.vi"("error in (no error)"=w559, "Hide passed/skiped?"=w551, "Test Tree In"=w561) -> ("error out"=w558:errorcluster, "Test Tree Out"=w560:refnum<class "Test Result Tree.lvclass">)  [unwired: 7 in]
        n222 = call "Update.vi"("error in (no error)"=w558, "Test Tree In"=w560) -> ("error out"=w556:errorcluster, "Test Tree Out"=w563:refnum<class "Test Result Tree.lvclass">)  [unwired: 8 in]
        n223 = Bundle By Name(cluster=w565, "Test Tree"=w563) -> (w564:refnum<class "Execution UI.lvclass">)
        n224 = Select(t="Showing only failed tests" ("Status"), s=w551, f="Showing all tests" ("Status")) -> (s? t:f=w554:string)
        n225 = call "Update Status.vi"("error in (no error)"=w556, "Status"=w554, "Execution UI In"=w564) -> ("error out"=w555:errorcluster, "Execution UI Out"=w557:refnum<class "Execution UI.lvclass">)  [unwired: 7 in]
      }
      frame "Open Front Panel" {
        n226 = Variant To Data(error in=w575, type="" ("Empty String Constant"), Variant=w574) -> (data=w569:string, error out=w570:errorcluster)
        n227 = call "Open Method Front Panel.vi"("error in (no error)"=w570, "String"=w569, "Execution UI In"=w568) -> ("error out"=w571:errorcluster, "Execution UI Out"=w572:refnum<class "Execution UI.lvclass">)  [unwired: 7 in]
      }
      frame "Update Description" {
        n228 = Variant To Data(error in=w584, type=string[] [], Variant=w583) -> (data=w581:string[], error out=w580:errorcluster)
        n229 = for {
          tunnel: w581 -> [w592] mode=indexing
          tunnel: w578 -> [w589]
          shift-right: [w590] -> w579
          shift-left: w580 -> [w591]
          shift-right: [w588] -> w576
          shift-left: "" ("Empty String Constant") -> [w587]
          w585 = "\r\n" ("End of Line Constant")
          n230 = Unbundle By Name(w589) -> ("Test Tree"=w593:refnum<class "Test Result Tree.lvclass">)
          n231 = call "Get Description.vi"("error in (no error)"=w591, "Tag"=w592, "Test Tree In"=w593) -> ("error out"=w590:errorcluster, "Description"=w586:string)  [unwired: 5 in, 2 out]
          n232 = Concatenate Strings(w587, w586, w585, w585) -> (w588:string)
        }
        "Description" <- w576
      }
      frame "Set Top Left Tree Node" {
        n233 = Variant To Data(error in=w603, type="", Variant=w601) -> (data=w598:string, error out=w595:errorcluster)
        n234 = Unbundle By Name(w602) -> ("Test Tree"=w599:refnum<class "Test Result Tree.lvclass">)
        n235 = call "Set Top Left Node.vi"("error in (no error)"=w595, "Test Class Qualified Name"=w598, "Test Tree in"=w599) -> ("error out"=w594:errorcluster, "Test Tree out"=w596:refnum<class "Test Result Tree.lvclass">)  [unwired: 7 in]
        n236 = Bundle By Name(cluster=w602, "Test Tree"=w596) -> (w597:refnum<class "Execution UI.lvclass">)
      }
      frame "Update Status" {
        n237 = Variant To Data(error in=w609, type="" ("Empty String Constant"), Variant=w608) -> (data=→"Status":string, error out=w605:errorcluster)
      }
      frame "Update Enable State" {
        n238 = Unbundle By Name(w617) -> ("Execution State"=w616:T4)
        n239 = case shown="\"Idle\"" w616 {
          tunnel: [T5."Enabled" ("Disabled") T5."Disabled and Grayed Out" ("Disabled")] -> w615
          tunnel: [T5."Disabled and Grayed Out" ("Disabled") T5."Enabled" ("Disabled")] -> w614
          tunnel: [T5."Disabled and Grayed Out" ("Disabled") T5."Enabled" ("Disabled")] -> w613
          tunnel: [T5."Disabled and Grayed Out" ("Disabled") T5."Enabled" ("Disabled")] -> w612
          tunnel: [T5."Disabled and Grayed Out" ("Disabled") T5."Enabled" ("Disabled")] -> w611
          tunnel: [T5."Disabled and Grayed Out" ("Disabled") T5."Enabled" ("Disabled")] -> w610
          frame "Running" {
          }
          frame "Idle" {
          }
        }
        n240 = property on="Stop" class="Bool"("DisabledEnum"=w615) -> ()  [unwired: 2 in, 2 out]
        n241 = property on="Run Single Test" class="Bool"("DisabledEnum"=w614) -> ()  [unwired: 2 in, 2 out]
        n242 = property on="Run All Tests" class="Bool"("DisabledEnum"=w613) -> ()  [unwired: 2 in, 2 out]
        n243 = property on="Refresh" class="Bool"("DisabledEnum"=w612) -> ()  [unwired: 2 in, 2 out]
        n244 = property on="Save" class="Bool"("DisabledEnum"=w611) -> ()  [unwired: 2 in, 2 out]
        n245 = property on="Eject" class="Bool"("DisabledEnum"=w610) -> ()  [unwired: 2 in, 2 out]
      }
      frame "Launch Results View" {
        n246 = vi-ref "Test Result View.lvclass:Result View.vi"() -> (w639:refnum<vi>)
        n247 = Unbundle By Name(w645) -> ("Test Tree"=w642:refnum<class "Test Result Tree.lvclass">, "Test Case Finder"=w632:refnum<class "Test Finder.lvclass">)
        n248 = property class="VI"(reference=w639, error in=w643) -> (error out=w634:errorcluster, "Path"=w638:path)  [unwired: 1 out]
        n249 = call "Read TestCase map.vi"("Test Finder In"=w632) -> ("TestCase map"=w631:map{string, map{string, path}})  [unwired: 8 in, 2 out]
        n250 = Open VI Reference(type specifier VI Refnum (for type only)=refnum<vi> refnum, vi path=w638, options=128, error in (no error)=w634) -> (vi reference=w635:refnum<vi>, error out=w637:errorcluster)  [unwired: 2 in]
        n251 = call-by-ref "Start Asynchronous Call"(reference=w635, error in=w637, "TestCase map"=w631, "Test Tree"=w642) -> (reference out=w640:refnum<vi>, error out=w641:errorcluster)  [unwired: 10 in]
        n252 = Close Reference(reference=w640, error in (no error)=w641) -> (error out=w644:errorcluster)
      }
      frame "Enable Execution Profiler" {
        n253 = Unbundle By Name(w664) -> ("Execution Profiler"=w649:refnum<class "Execution Profiler.lvclass">, "Result Collector"=w660:refnum<class "Result Collector.lvclass">, "Test Case Finder"=w655:refnum<class "Test Finder.lvclass">)
        n254 = call-dynamic "Init.vi"("error in (no error)"=w647, "Process In"=w649) -> ("error out"=w648:errorcluster, "Process Out"=w646:refnum<class "Execution Profiler.lvclass">)  [unwired: 8 in]
        n255 = call "Set Result Collector.vi"("error in (no error)"=w648, "Result Collector In"=w660, "Execution Profiler In"=w646) -> ("error out"=w658:errorcluster, "Execution Profiler Out"=w659:refnum<class "Execution Profiler.lvclass">)  [unwired: 7 in]
        n256 = call "Set Test Finder.vi"("error in (no error)"=w658, "Test Finder"=w655, "Execution Profiler In"=w659) -> ("error out"=w656:errorcluster, "Execution Profiler Out"=w657:refnum<class "Execution Profiler.lvclass">)  [unwired: 7 in]
        n257 = call "Start.vi"("error in (no error)"=w656, "Process In"=w657) -> ("error out"=w661:errorcluster, "Process Out"=w653:refnum<class "Execution Profiler.lvclass">)  [unwired: 8 in]
        n258 = Current VI's Menubar() -> (w652:refnum<k9>)
        n259 = Bundle By Name(cluster=w664, "Execution Profiler"=w653) -> (w654:refnum<class "Execution UI.lvclass">)
        n260 = Set Menu Item Info(6:TRUE ("checked"), 7:"Execution Profiler...", 11:w652) -> ()  [unwired: 4 in, 2 out]
        n261 = call "Update Status.vi"("error in (no error)"=w661, "Status"="Run a test to generate an execution analysis.", "Execution UI In"=w654) -> ("error out"=w663:errorcluster, "Execution UI Out"=w662:refnum<class "Execution UI.lvclass">)  [unwired: 7 in]
      }
      frame "Enable Coverage Analyzer" {
        n262 = Unbundle By Name(w681) -> ("Coverage Analyzer"=w667:refnum<class "Coverage Analyzer Process.lvclass">, "Result Collector"=w676:refnum<class "Result Collector.lvclass">)
        n263 = call-dynamic "Init.vi"("error in (no error)"=w677, "Process In"=w667) -> ("error out"=w668:errorcluster, "Process Out"=w666:refnum<class "Coverage Analyzer Process.lvclass">)  [unwired: 8 in]
        n264 = call "Set Result Collector.vi"("error in (no error)"=w668, "Result Collector In"=w676, "Coverage Analyzer Process in"=w666) -> ("error out"=w669:errorcluster, "Coverage Analyzer Process out"=w670:refnum<class "Coverage Analyzer Process.lvclass">)  [unwired: 7 in]
        n265 = call "Start.vi"("error in (no error)"=w669, "Process In"=w670) -> ("error out"=w678:errorcluster, "Process Out"=w674:refnum<class "Coverage Analyzer Process.lvclass">)  [unwired: 8 in]
        n266 = Current VI's Menubar() -> (w673:refnum<k9>)
        n267 = Bundle By Name(cluster=w681, "Coverage Analyzer"=w674) -> (w675:refnum<class "Execution UI.lvclass">)
        n268 = Set Menu Item Info(6:TRUE ("checked"), 7:"Coverage Analyzer...", 11:w673) -> ()  [unwired: 4 in, 2 out]
        n269 = call "Update Status.vi"("error in (no error)"=w678, "Status"="Run a test to generate coverage analysis...", "Execution UI In"=w675) -> ("error out"=w680:errorcluster, "Execution UI Out"=w679:refnum<class "Execution UI.lvclass">)  [unwired: 7 in]
      }
      frame "Disable Execution Profiler" {
        n270 = Unbundle By Name(w695) -> ("Execution Profiler"=w691:refnum<class "Execution Profiler.lvclass">)
        n271 = call-dynamic "Stop.vi"("error in (no error)"=w690, "Process In"=w691) -> ("error out"=w692:errorcluster, "Process Out"=w684:refnum<class "Execution Profiler.lvclass">)  [unwired: 7 in, 1 out]
        n272 = call-dynamic "Clear.vi"("error in (no error)"=w692, "Process In"=w684) -> ("error out"=w685:errorcluster, "Process Out"=w683:refnum<class "Execution Profiler.lvclass">)  [unwired: 8 in]
        n273 = Bundle By Name(cluster=w695, "Execution Profiler"=w683) -> (w689:refnum<class "Execution UI.lvclass">)
        n274 = Current VI's Menubar() -> (w688:refnum<k9>)
        n275 = call "Update Status.vi"("error in (no error)"=w685, "Status"="Execution profiler disabled.", "Execution UI In"=w689) -> ("error out"=w694:errorcluster, "Execution UI Out"=w693:refnum<class "Execution UI.lvclass">)  [unwired: 7 in]
        n276 = Set Menu Item Info(6:FALSE ("checked"), 7:"Execution Profiler...", 11:w688) -> ()  [unwired: 4 in, 2 out]
      }
      frame "Disable Coverage Analyzer" {
        n277 = Unbundle By Name(w709) -> ("Coverage Analyzer"=w705:refnum<class "Coverage Analyzer Process.lvclass">)
        n278 = call-dynamic "Stop.vi"("error in (no error)"=w704, "Process In"=w705) -> ("error out"=w706:errorcluster, "Process Out"=w698:refnum<class "Coverage Analyzer Process.lvclass">)  [unwired: 7 in, 1 out]
        n279 = call-dynamic "Clear.vi"("error in (no error)"=w706, "Process In"=w698) -> ("error out"=w699:errorcluster, "Process Out"=w697:refnum<class "Coverage Analyzer Process.lvclass">)  [unwired: 8 in]
        n280 = Bundle By Name(cluster=w709, "Coverage Analyzer"=w697) -> (w703:refnum<class "Execution UI.lvclass">)
        n281 = Current VI's Menubar() -> (w702:refnum<k9>)
        n282 = call "Update Status.vi"("error in (no error)"=w699, "Status"="Coverage analyzer disabled.", "Execution UI In"=w703) -> ("error out"=w708:errorcluster, "Execution UI Out"=w707:refnum<class "Execution UI.lvclass">)  [unwired: 7 in]
        n283 = Set Menu Item Info(6:FALSE ("checked"), 7:"Coverage Analyzer...", 11:w702) -> ()  [unwired: 4 in, 2 out]
      }
      frame "Stop" {
        n284 = call "Enqueue Message.vi"("error in (no error)"=w716, "Message"="Exit", "Process In"=w715) -> ("error out"=w717:errorcluster, "Process Out"=w713:refnum<class "Execution UI.lvclass">)  [unwired: 7 in]
        n285 = call "Stop Processes.vi"("error in (no error)"=w717, "Execution UI In"=w713) -> ("error out"=w711:errorcluster, "Execution UI Out"=w712:refnum<class "Execution UI.lvclass">)  [unwired: 8 in]
      }
      frame "Exit" {
        n286 = control-ref of="This VI"() -> (w722:refnum<vi>)
        n287 = invoke on="Invoke Node" class="VI" method="FP.Close"(reference=w722, error in=w718) -> (reference out=w720:refnum<vi>, error out=w721:errorcluster)  [unwired: 1 in, 1 out]
        n288 = Close Reference(reference=w720, error in (no error)=w721) -> (error out=w719:errorcluster)
        n289 = call "Finish.vi"("error in (no error)"=w719, "Process In"=w724) -> ("error out"=w723:errorcluster, "Process Out"=w725:refnum<class "Execution UI.lvclass">)  [unwired: 8 in]
        n290 = call-dynamic "Clear.vi"("error in (no error)"=w723, "Execution UI In"=w725) -> ("error out"=w727:errorcluster, "Execution UI Out"=w728:refnum<class "Execution UI.lvclass">)  [unwired: 8 in]
      }
    }
    n291 = call "Handle Process Errors.vi"("error in (no error)"=w328, "Process In"=w334) -> ("error out"=w329:errorcluster, "Process Out"=w330:refnum<class "Execution UI.lvclass">)  [unwired: 8 in]
  }
  n292 = Unregister For Events(event registration refnum=w13, error in=w6) -> (error out=w4:errorcluster)
  n293 = Merge Errors(w4, w10) -> (→"error out":errorcluster)
